vi "P612.vi"(4 "Special Function In":string, 6 "Velocity":dbl, 7 "Abort":refnum<vi>, 8 "Axis":bool[](array[boolean]), 9 "Positions":dbl[](array[numeric]), 10 "Action":T1=enum."MVR", 11 "VISA In":refnum<visa-resource-name>) -> (0 "Special Function":string, 1 "Status":bool, 2 "Position Out":dbl[](array[numeric]), 3 "VISA Out":refnum<visa-resource-name>)   [LabVIEW 2014]
uses:
  Controls/StageStates.ctl
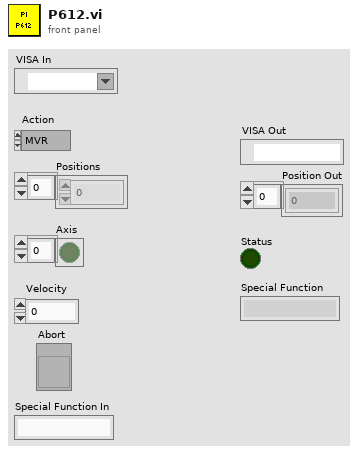
[diagram p1: front panel]
types:
  T1 = typedef "StageStates.ctl" = enum16{"POSITION", "MVR", "MOVE", "HALT", "ONTARGET", "ERROR", "EXIT", "HOME", "ZEROPOS", "NANOPOS", "QUIT", "ANALOG"}
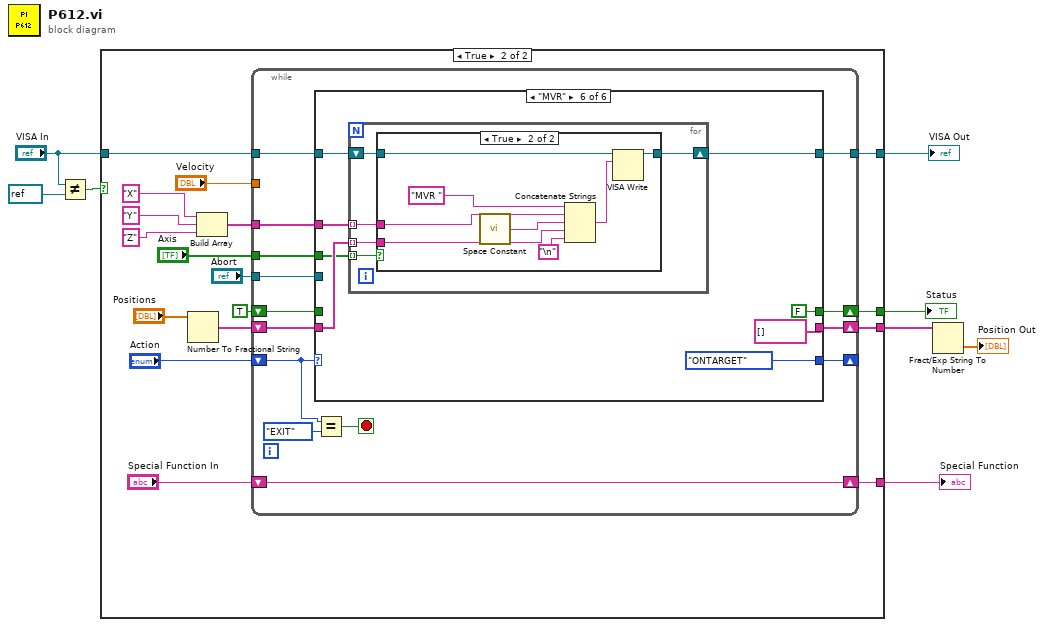
[diagram p0: block diagram]
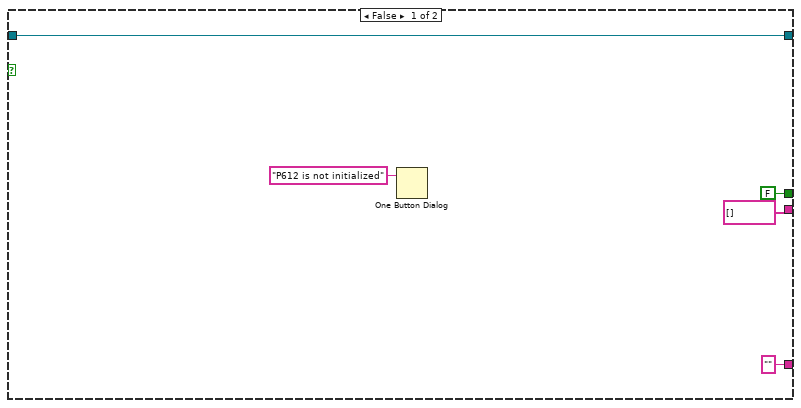
[diagram p2: hidden frame]
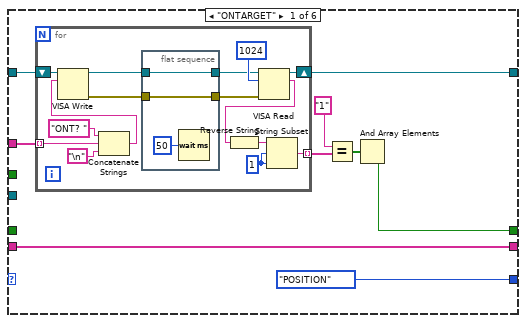
[diagram p3: hidden frame]
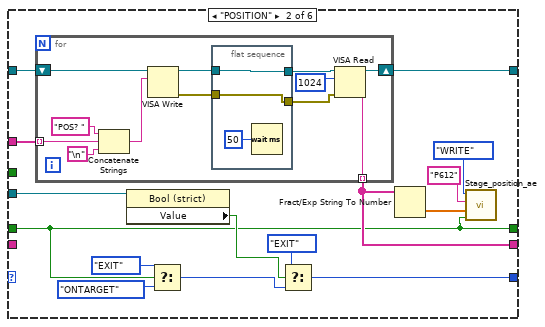
[diagram p4: hidden frame]
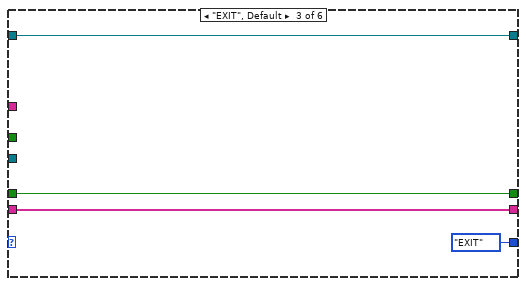
[diagram p5: hidden frame]
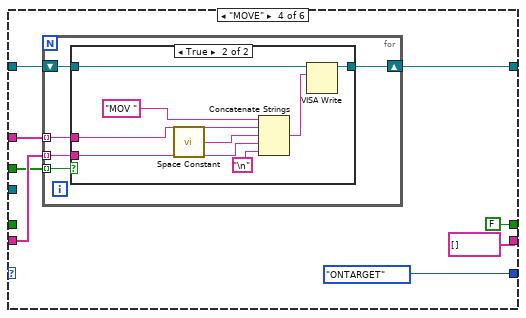
[diagram p6: hidden frame]
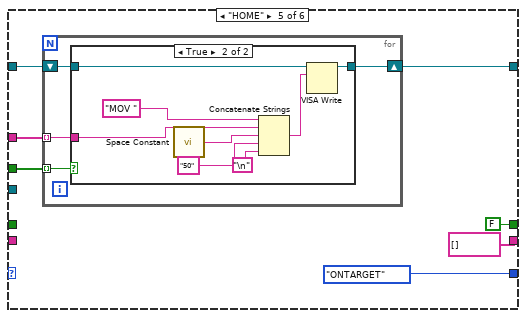
[diagram p8: hidden frame]
diagram:
  n1 = Not Equal?(x="VISA In", y=refnum<visa-resource-name> refnum ("VISA In")) -> (x != y?=w8:bool)
  n2 = case shown="True" w8 {
    tunnel: "VISA In" -> [w12 w30]
    tunnel: [w12 w19] -> w5
    tunnel: [FALSE w18] -> w3
    tunnel: [string[] [] w17] -> w2
    tunnel: ["" ("Special Function In") w16] -> w1
    frame False {
      n3 = One Button Dialog(message="P612 is not initialized") -> ()  [unwired: 1 in, 1 out]
    }
    frame True {
      n4 = Number To Fractional String(number="Positions") -> (F-format string=w23:string[])  [unwired: 3 in]
      n5 = Build Array("X", "Y", "Z") -> (w26:string[])
      n6 = while {
        tunnel: w26 -> [w44]
        tunnel: w30 -> [w43]
        shift-right: [w35] -> _
        shift-left: "Action" -> [w38]
        shift-right: [w41] -> w17
        shift-left: w23 -> [w42]
        shift-right: [w39] -> w18
        shift-left: TRUE -> [w40]
        tunnel: "Axis" -> [w37]
        shift-right: [w34] -> w16
        shift-left: "Special Function In" -> [w34]
        tunnel: "Velocity" -> [_]
        tunnel: [w33] -> w19
        tunnel: "Abort" -> [w31]
        stop <- w32 stop-if-true
        n7 = case shown="\"MVR\"" w38 {
          tunnel: w44 -> [w53 w86 _ w113 w134 w155]
          tunnel: w43 -> [w47 w85 w105 w112 w133 w154]
          tunnel: w42 -> [w49 _ w103 w111 _ w153]
          tunnel: [w49 w75 w103 string[] [] string[] [] string[] []] -> w41
          tunnel: w40 -> [_ w72 w104 _ _ _]
          tunnel: [w48 w72 w104 FALSE FALSE FALSE] -> w39
          tunnel: w37 -> [_ _ _ w110 w132 w152]
          tunnel: [StageStates."POSITION" ("Action") w80 StageStates."EXIT" ("Action") StageStates."ONTARGET" ("Action") StageStates."ONTARGET" ("Action") StageStates."ONTARGET" ("Action")] -> w35
          tunnel: [w46 w79 w105 w108 w130 w150] -> w33
          tunnel: w31 -> [_ w73 _ _ _ _]
          frame "ONTARGET" {
            n8 = for {
              tunnel: w53 -> [w68] mode=indexing
              tunnel: [w67] -> w52 mode=indexing
              shift-right: [w58] -> w46
              shift-left: w47 -> [w59]
              w62 = 1 ("length (rest)")
              n9 = Concatenate Strings("ONT? " ("string"), w68, "\n") -> (w61:string)
              n10 = VISA Write(VISA resource name=w59, write buffer=w61) -> (VISA resource name out=w57:refnum<visa-resource-name>, error out=w54:errorcluster)  [unwired: 1 in, 1 out]
              n11 = flat-sequence {
                tunnel: w57 -> [w70]
                tunnel: [w70] -> w56
                tunnel: [w69] -> w55
                tunnel: w54 -> [w69]
                frame #0 {
                  n12 = Wait (ms)(milliseconds to wait=u32 50) -> ()  [unwired: 1 out]
                }
              }
              n13 = VISA Read(VISA resource name=w56, byte count=u32 1024, error in (no error)=w55) -> (VISA resource name out=w58:refnum<visa-resource-name>, read buffer=w60:string)  [unwired: 2 out]
              n14 = Reverse String(1:w60) -> (0:w63:string)
              n15 = String Subset(string=w63, offset (0)=w62, length (rest)=w62) -> (substring=w67:string)
            }
            n16 = Equal?(x="1", y=w52) -> (x = y?=w50:bool[])
            n17 = And Array Elements(Boolean array=w50) -> (logical AND=w48:bool)
          }
          frame "POSITION" {
            n18 = for {
              tunnel: w86 -> [w98] mode=indexing
              tunnel: [w92] -> w75 mode=indexing
              shift-right: [w87] -> w79
              shift-left: w85 -> [w93]
              n19 = Concatenate Strings("POS? " ("string"), w98, "\n") -> (w94:string)
              n20 = VISA Write(VISA resource name=w93, write buffer=w94) -> (VISA resource name out=w90:refnum<visa-resource-name>, error out=w88:errorcluster)  [unwired: 1 in, 1 out]
              n21 = flat-sequence {
                tunnel: [w101] -> w91
                tunnel: w90 -> [w101]
                tunnel: [w100] -> w89
                tunnel: w88 -> [w100]
                frame #0 {
                  n22 = Wait (ms)(milliseconds to wait=u32 50) -> ()  [unwired: 1 out]
                }
              }
              n23 = VISA Read(VISA resource name=w91, byte count=u32 1024, error in (no error)=w89) -> (VISA resource name out=w87:refnum<visa-resource-name>, read buffer=w92:string)  [unwired: 2 out]
            }
            n24 = property class="Bool (strict)"(reference=w73) -> ("Value"=w74:bool)  [unwired: 1 in, 2 out]
            n25 = Select(t=StageStates."EXIT" ("Action"), s=w72, f=StageStates."ONTARGET" ("Action")) -> (s? t:f=w83:T1)
            n26 = Select(t=StageStates."EXIT", s=w74, f=w83) -> (s? t:f=w80:T1)
            n27 = Fract/Exp String To Number(string=w75) -> (number=w78:dbl[])  [unwired: 3 in, 1 out]
            n28 = call "Stage_position_ae.vi"("Status In"=w72, "Position In"=w78, "StageID"="P612", "Enum"=enum16{"WRITE", "READ"}."WRITE") -> ()  [unwired: 6 in, 2 out]
          }
          frame "EXIT", Default {
          }
          frame "MOVE" {
            n29 = for {
              tunnel: w113 -> [w118] mode=indexing
              tunnel: w111 -> [w117] mode=indexing
              shift-right: [w115] -> w108
              shift-left: w112 -> [w116]
              tunnel: w110 -> [w114] mode=indexing
              n30 = case shown="True" w114 {
                tunnel: w118 -> [_ w125]
                tunnel: w117 -> [_ w122]
                tunnel: w116 -> [w119 w121]
                tunnel: [w119 w120] -> w115
                frame False {
                }
                frame True {
                  n31 = call <vilib>:"Space Constant.vi"() -> ("String"=w123:string)
                  n32 = Concatenate Strings("MOV ", w125, w123, w122, "\n") -> (w127:string)
                  n33 = VISA Write(VISA resource name=w121, write buffer=w127) -> (VISA resource name out=w120:refnum<visa-resource-name>)  [unwired: 1 in, 2 out]
                }
              }
            }
          }
          frame "HOME" {
            n34 = for {
              tunnel: w134 -> [w138] mode=indexing
              shift-right: [w136] -> w130
              shift-left: w133 -> [w137]
              tunnel: w132 -> [w135] mode=indexing
              n35 = case shown="True" w135 {
                tunnel: w138 -> [_ w145]
                tunnel: w137 -> [w139 w142]
                tunnel: [w139 w141] -> w136
                frame False {
                }
                frame True {
                  n36 = call <vilib>:"Space Constant.vi"() -> ("String"=w143:string)
                  n37 = Concatenate Strings("MOV ", w145, w143, "50" ("string"), "\n") -> (w147:string)
                  n38 = VISA Write(VISA resource name=w142, write buffer=w147) -> (VISA resource name out=w141:refnum<visa-resource-name>)  [unwired: 1 in, 2 out]
                }
              }
            }
          }
          frame "MVR" {
            n39 = for {
              tunnel: w155 -> [w160] mode=indexing
              tunnel: w153 -> [w159] mode=indexing
              shift-right: [w157] -> w150
              shift-left: w154 -> [w158]
              tunnel: w152 -> [w156] mode=indexing
              n40 = case shown="True" w156 {
                tunnel: w160 -> [_ w167]
                tunnel: w159 -> [_ w164]
                tunnel: w158 -> [w161 w163]
                tunnel: [w161 w162] -> w157
                frame False {
                }
                frame True {
                  n41 = call <vilib>:"Space Constant.vi"() -> ("String"=w165:string)
                  n42 = Concatenate Strings("MVR ", w167, w165, w164, "\n") -> (w169:string)
                  n43 = VISA Write(VISA resource name=w163, write buffer=w169) -> (VISA resource name out=w162:refnum<visa-resource-name>)  [unwired: 1 in, 2 out]
                }
              }
            }
          }
        }
        n44 = Equal?(x=w38, y=StageStates."EXIT") -> (x = y?=w32:bool)
      }
    }
  }
  "VISA Out" <- w5
  "Status" <- w3
  "Special Function" <- w1
  n45 = Fract/Exp String To Number(string=w2) -> (number=→"Position Out":dbl[])  [unwired: 3 in, 1 out]
